vi "Unflatten.vi"(8 "error in (no error)":errorcluster, 10 "JSON stream":string, 11 "JSON Value in":refnum<class "JSON Value.lvclass">) -> (0 "error out":errorcluster, 1 "Empty?":bool, 2 "rest of JSON stream":string, 3 "JSON Value out":refnum<class "JSON Value.lvclass">)   [LabVIEW 2020, in "Library Commun.lvlib" / "JSON Value.lvclass"]
doc: "Converts a <b>JSON stream</b> into a <b>JSON Value</b>.\n\nCopyright 2012 James David Powell, Shaun Rumbell and Ton Plomp\nMore information on http://lavag.org/topic/16217-cr-json-labview"
uses:
  JSON Value.lvclass
  JSON Array/JSON Array.lvclass
  C:/Users/ngarcin/OneDrive - Altyor/Standard TB/Class/JSON API/JSON Value/JSON Value.lvclass
  JSON Object/JSON Object.lvclass
  JSON Scalar/JSON Scalar.lvclass
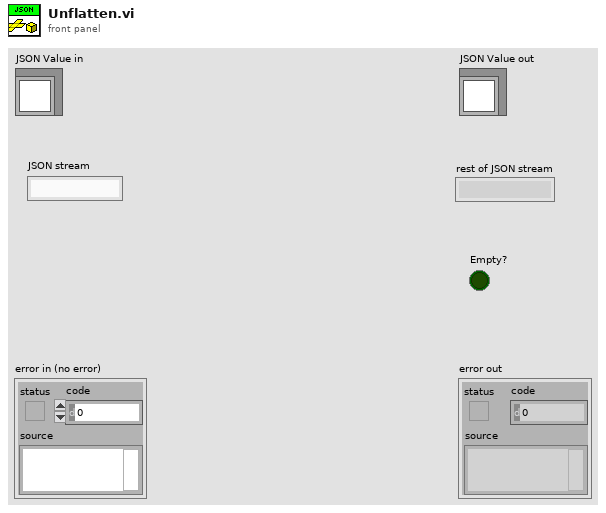
[diagram p1: front panel]
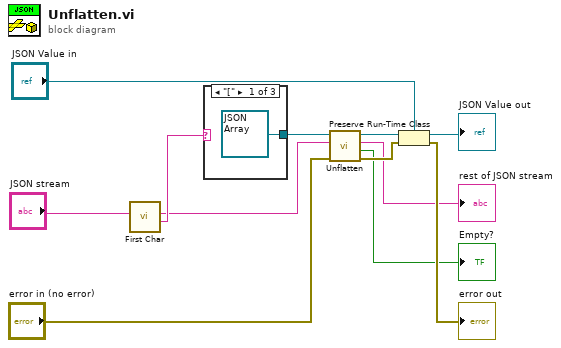
[diagram p0: block diagram]
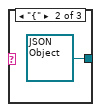
[diagram p2: hidden frame]
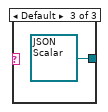
[diagram p3: hidden frame]
diagram:
  n1 = call "First Char.vi"("String in"="JSON stream") -> ("First Char"=w11:string, "String"=w2:string)  [unwired: 9 in]
  n2 = case shown="\"[\"" w11 {
    tunnel: [refnum<class "JSON Array.lvclass"> refnum ("JSON Array.lvclass") refnum<class "JSON Object.lvclass"> refnum ("JSON Object.lvclass") refnum<class "JSON Scalar.lvclass"> refnum ("JSON Scalar.lvclass")] -> w7
    frame "[" {
    }
    frame "{" {
    }
    frame Default {
    }
  }
  n3 = call-dynamic "Unflatten.vi"("error in (no error)"="error in (no error)", "JSON stream"=w2, "JSON Value in"=w7) -> ("error out"=w6:errorcluster, "Empty?"=→"Empty?":bool, "rest of JSON stream"=→"rest of JSON stream":string, "JSON Value out"=w5:refnum<class "JSON Value.lvclass">)  [unwired: 5 in]
  n4 = Preserve Run-Time Class(object in=w5, error in=w6, 2:"JSON Value in") -> (object out=→"JSON Value out":refnum<class "JSON Value.lvclass">, error out=→"error out":errorcluster)
